vi "broadcastReg-Test1.vi"() -> ()   [LabVIEW 2017]
uses:
  user.lib/_NEVSTOP/Communicable State Machine(CSM)/_Support/Common/Trim Single line Text.vi
  user.lib/_NEVSTOP/Communicable State Machine(CSM)/_Support/BroadcastRegistry/BroadcastRegistry.lvclass
  user.lib/_NEVSTOP/Communicable State Machine(CSM)/Communicable State Machine.lvlib
panel:
  out "Registry":variant
  out "Response Message Info":string[](array[string])
  in  "Boolean":bool
  in  "scripts":string="status@source >> api@target -><register>\nstatus@source >> api2@target -><register>"
  in  "Target":string="target"
  in  "Source":string="source"
  in  "Status":string="status"
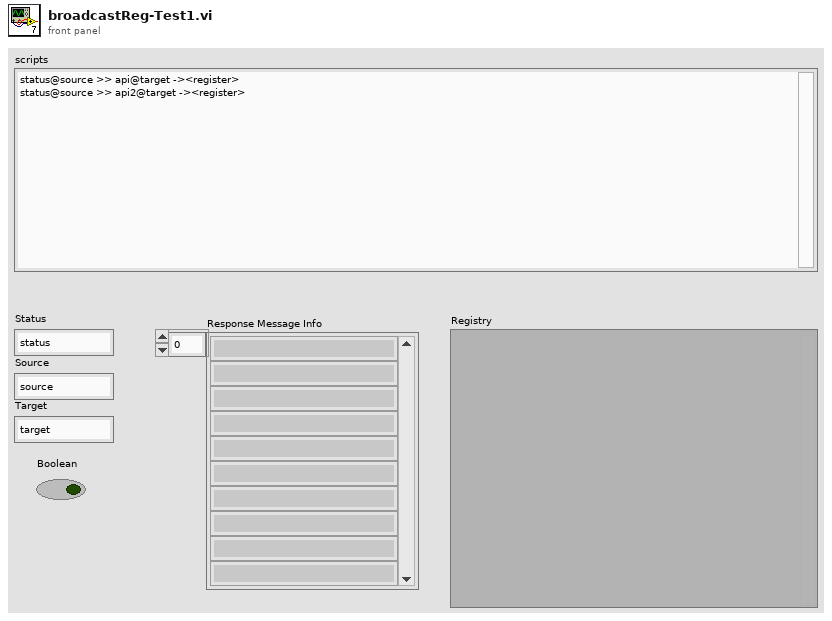
[diagram p1: front panel]
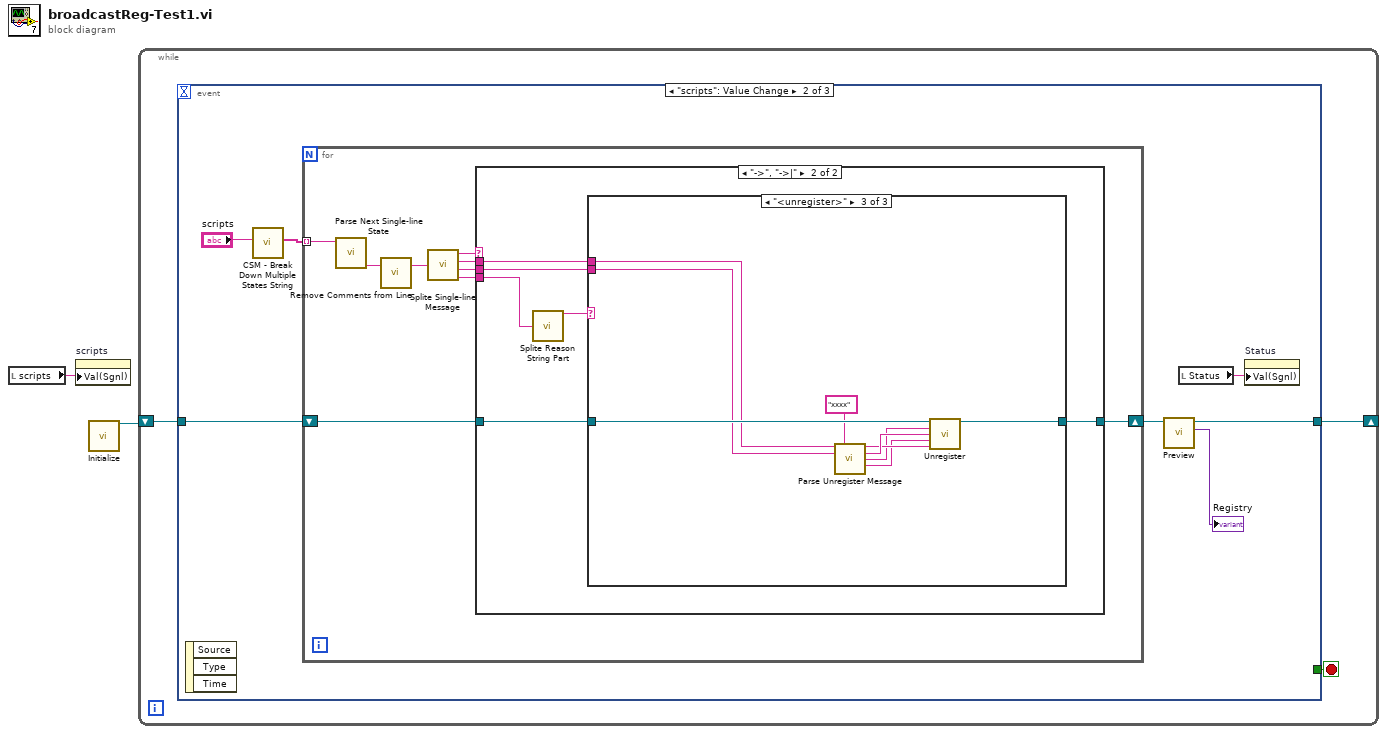
[diagram p0: block diagram]
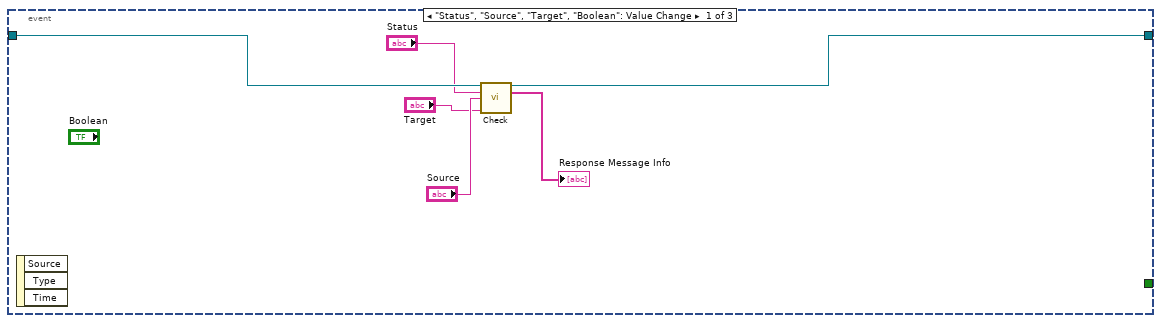
[diagram p2: hidden frame]
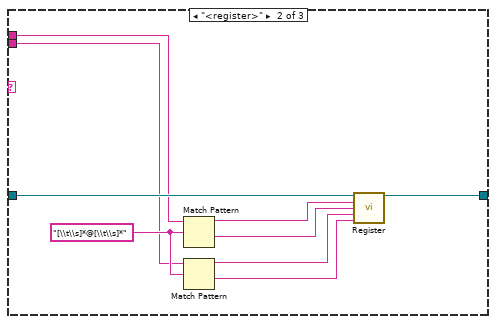
[diagram p5: hidden frame]
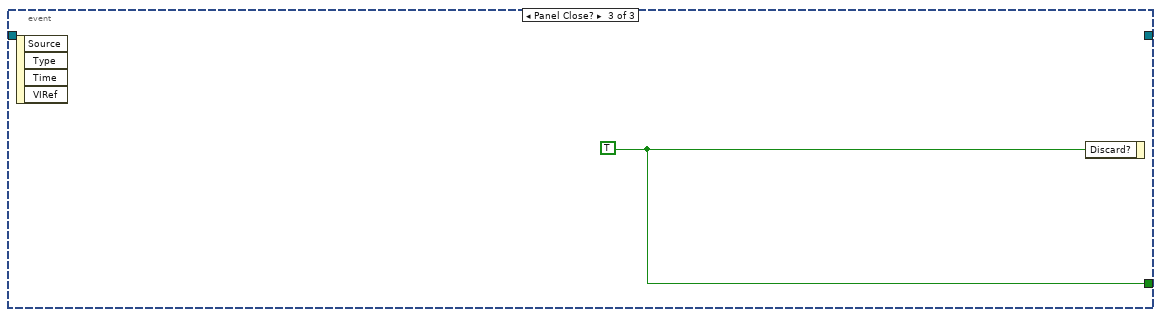
[diagram p6: hidden frame]
diagram:
  n1 = local read "scripts"() -> (w1:string)
  n2 = property on="scripts" class="Str"("Val(Sgnl)"=w1) -> ()  [unwired: 2 in, 2 out]
  n3 = call "Initialize.vi"() -> ("BroadcastRegistry out"=w2:refnum<class "BroadcastRegistry.lvclass">)  [unwired: 15 in]
  n4 = while {
    shift-right: [w3] -> _
    shift-left: w2 -> [w5]
    stop <- w4 stop-if-true
    n5 = event shown="[1] \"scripts\": Value Change" {
      selector: _ -> [_ _ _]
      dyn-events: _ -> [_ _ _]
      timeout: _ -> [_ _ _]
      tunnel: w5 -> [w11 w15 _]
      tunnel: [_ _ w54] -> w4
      tunnel: [w6 w14 _] -> w3
      event "Status", "Source", "Target", "Boolean": Value Change {
        n6 = event-data() -> ()  [unwired: 1 in, 3 out]
        n7 = call "Check.vi"("BroadcastRegistry in"=w11, "Status"="Status", "Source"="Source", "Target"="Target") -> ("BroadcastRegistry out"=w6:refnum<class "BroadcastRegistry.lvclass">, "Response Message Info"=→"Response Message Info":string[])  [unwired: 10 in]
      }
      event "scripts": Value Change {
        n8 = event-data() -> ()  [unwired: 1 in, 3 out]
        n9 = call "CSM - Break Down Multiple States String.vi"("States"="scripts") -> ("Multiple States"=w18:string[])  [unwired: 10 in]
        n10 = for {
          tunnel: w18 -> [w25] mode=indexing
          shift-right: [w19] -> w16
          shift-left: w15 -> [w20]
          n11 = call "Parse Next Single-line State.vi"("States Queue"=w25) -> ("Next Single-line State"=w26:string)  [unwired: 9 in, 1 out]
          n12 = call "Remove Comments from Line.vi"("single-line text"=w26) -> ("single-line text without comments"=w27:string)  [unwired: 2 in]
          n13 = call "Splite Single-line Message.vi"("single-line text"=w27) -> ("operator"=w24:string, "state"=w23:string, "args"=w22:string, "source/target"=w21:string)  [unwired: 6 in]
          n14 = case shown="\"->\", \"->|\"" w24 {
            tunnel: w23 -> [_ w34]
            tunnel: w22 -> [_ w33]
            tunnel: w21 -> [_ w30]
            tunnel: w20 -> [w28 w32]
            tunnel: [w28 w31] -> w19
            frame "False", Default {
            }
            frame "->", "->|" {
              n15 = call "Splite Reason String Part.vi"("Single-line -& Reason"=w30) -> ("CSM Name"=w29:string)  [unwired: 12 in, 2 out]
              n16 = case shown="\"<unregister>\"" w29 {
                tunnel: w34 -> [_ w41 w51]
                tunnel: w33 -> [_ w40 w50]
                tunnel: w32 -> [w35 w44 w53]
                tunnel: [w35 w43 w52] -> w31
                frame "False", Default {
                }
                frame "<register>" {
                  w42 = "[\\t\\s]*@[\\t\\s]*" ("regular expression")
                  n17 = Match Pattern(string=w41, regular expression=w42) -> (before substring=w36:string, after substring=w37:string)  [unwired: 1 in, 2 out]
                  n18 = Match Pattern(string=w40, regular expression=w42) -> (before substring=w38:string, after substring=w39:string)  [unwired: 1 in, 2 out]
                  n19 = call "Register.vi"("BroadcastRegistry in"=w44, "status"=w36, "source"=w37, "api"=w38, "target"=w39) -> ("BroadcastRegistry out"=w43:refnum<class "BroadcastRegistry.lvclass">)  [unwired: 10 in]
                }
                frame "<unregister>" {
                  n20 = call "Parse Unregister Message.vi"("state"=w51, "Module Name"="xxxx", "args"=w50) -> ("target"=w47:string, "source"=w48:string, "status"=w45:string, "api"=w46:string)  [unwired: 9 in]
                  n21 = call "Unregister.vi"("BroadcastRegistry in"=w53, "Status"=w45, "Source"=w48, "api"=w46, "Target"=w47) -> ("BroadcastRegistry out"=w52:refnum<class "BroadcastRegistry.lvclass">)  [unwired: 10 in]
                }
              }
            }
          }
        }
        n22 = call "Preview.vi"("BroadcastRegistry in"=w16) -> ("Registry"=→"Registry":variant, "BroadcastRegistry out"=w14:refnum<class "BroadcastRegistry.lvclass">)  [unwired: 8 in, 1 out]
        n23 = local read "Status"() -> (w12:string)
        n24 = property on="Status" class="Str"("Val(Sgnl)"=w12) -> ()  [unwired: 2 in, 2 out]
      }
      event Panel Close? {
        w54 = TRUE ("Discard?")
        n25 = event-data() -> ()  [unwired: 1 in, 4 out]
        n26 = event-data("Discard?"=w54) -> ()  [unwired: 1 in, 1 out]
      }
    }
  }
